vi "DAQmx Timing (Change Detection).vi"(0 "task/channels in":refnum<k21>, 1 "sample mode":i32(ring)=10178 items=["Finite Samples"=10178, "Continuous Samples"=10123, "Hardware Timed Single Point"=12522], 2 "samples per channel":i32=1000, 7 "rising edge physical channels":tag, 9 "falling edge physical channels":tag, 11 "error in":errorcluster) -> (4 "task out":refnum<k21>, 15 "error out":errorcluster)   [LabVIEW 2011]
doc: "Configures the task to acquire samples on the rising and/or falling edges of the lines or ports you specify. To detect both rising and falling edges on a line or port, wire the name of that line or port to both <B>rising edge physical channels</B> and <B>falling edge physical channels</B>."
uses:
  C:/Program Files/National Instruments/LabVIEW 2011/resource/objmgr/daqmx.rc
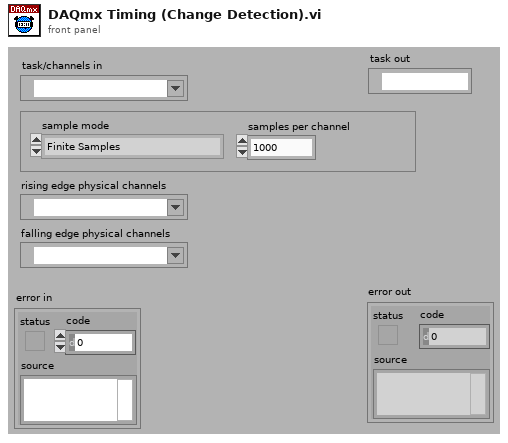
[diagram p1: front panel]
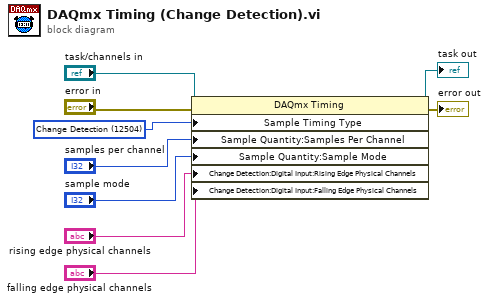
[diagram p0: block diagram]
diagram:
  w3 = 12504 items=["Sample Clock"=10388, "Handshake"=10389, "Implicit"=10451, "On Demand"=10390, "Change Detection"=12504] ("Sample Timing Type")
  n1 = property class="DAQmx Timing"(reference="task/channels in", error in="error in", "Sample Timing Type"=w3, "Sample Quantity:Samples Per Channel"="samples per channel", "Sample Quantity:Sample Mode"="sample mode", "Change Detection:Digital Input:Rising Edge Physical Channels"="rising edge physical channels", "Change Detection:Digital Input:Falling Edge Physical Channels"="falling edge physical channels") -> (reference out=→"task out":refnum<k21>, error out=→"error out":errorcluster)
